vi "Initialize.vi"(7 "Serial Configuration":T1={"Baud Rate"=9600, "Parity"=0, "Data Bits"=8, "Stop Bits"=10, "Flow Control"=0} {"Flow Control" items=["None", "XON/XOFF", "RTS/CTS", "XON/XOFF & RTS/CTS", "DTR/DSR", "XON/XOFF & DTR/DSR"]; "Stop Bits" items=["1.0"=10, "1.5"=15, "2.0"=20]; "Data Bits" items=["7"=7, "8"=8]; "Parity" items=["None", "Odd", "Even", "Mark", "Space"]; "Baud Rate" items=["300"=300, "600"=600, "1200"=1200, "2400"=2400, "4800"=4800, "9600"=9600, "19200"=19200]}, 8 "error in (no error)":errorcluster, 9 "Reset (True)":bool=TRUE, 10 "ID Query (True)":bool=TRUE, 11 "VISA resource name":refnum<visa-resource-name>) -> (0 "error out":errorcluster, 3 "VISA resource name out":refnum<visa-resource-name>)   [LabVIEW 2012, in "ValveController.lvlib"]
doc: "Establishes communication with the instrument and optionally performs an instrument identification query and/or an instrument reset. It also places the instrument in a default state needed for other instrument driver operations. Therefore, call this VI before calling other instrument driver VIs for this instrument. Generally, you need to call the Initialize VI only once at the beginning of an application."
uses:
  <instrlib>/ValveController/ValveController.lvlib
panel:
  # "(c) 2007 <Enter Company Name Here>.  ALL RIGHTS RESERVED."
  # "EDIT: Change control description to remove example text for buses not supported."
  # "EDIT: Serial settings must match those on the physical instrument.  Review user's manual to determine the correct Flow Control protocol for the instrument.  \"None\" is the least robust option for this setting, and could lead to unreliable data transmission."
  # "EDIT: If your instrument does not support ID query or Reset, remove the ID Query or Reset control from the front panel and delete the case structure with the ID Query or Reset code from the block diagram."
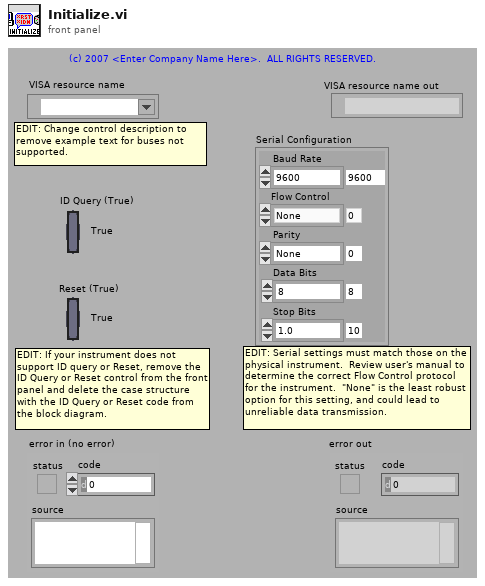
[diagram p1: front panel]
types:
  T1 = cluster{"Baud Rate":u32, "Parity":u16, "Data Bits":u16, "Stop Bits":u16, "Flow Control":u16}
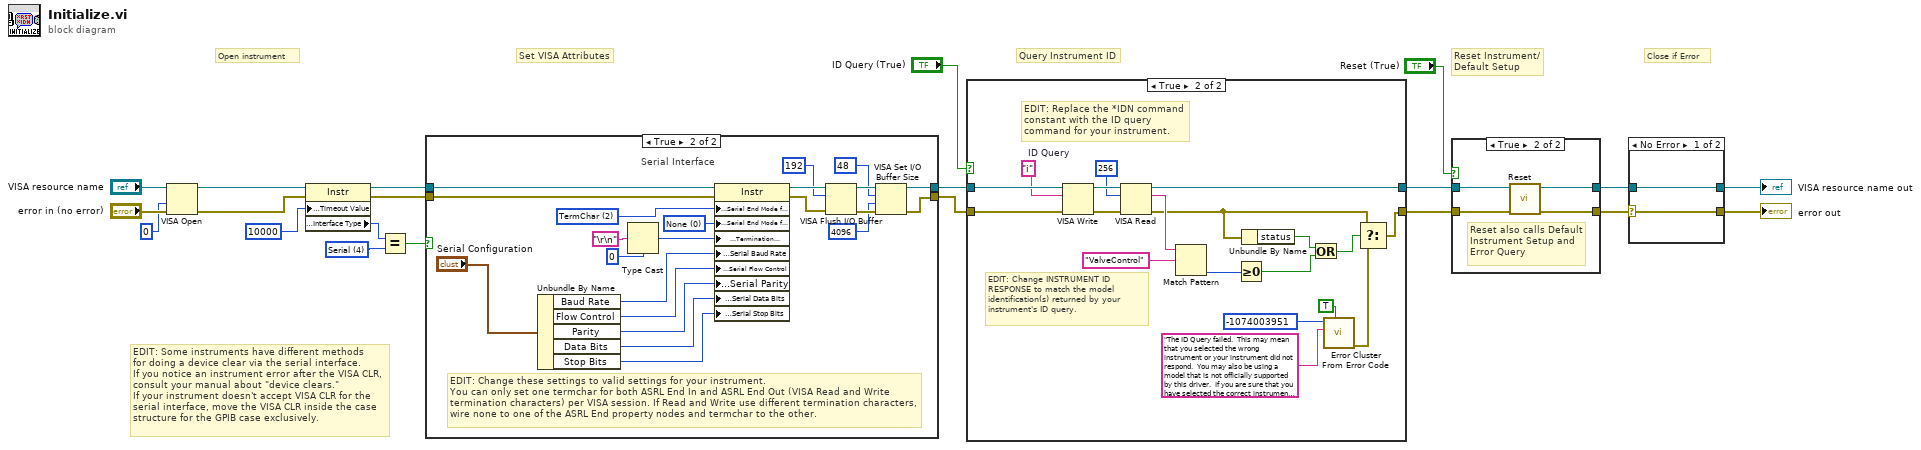
[diagram p0: block diagram]
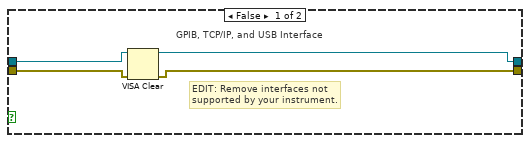
[diagram p2: hidden frame]
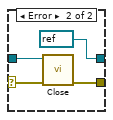
[diagram p3: hidden frame]
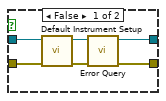
[diagram p4: hidden frame]
diagram:
  w8 = u16 4 items=["GPIB"=1, "VXI"=2, "GPIB-VXI"=3, "Serial"=4, "PXI"=5, "TCPIP"=6, "USB"=7] ("Interface Information:Interface Type")
  # "EDIT: Some instruments have different methods\nfor doing a device clear via the serial interface.  \nIf you notice an instrument error after the VISA CLR,\nconsult your manual about \"device clears.\"  \nIf your instrument doesn't accept VISA CLR for the\nserial interface, move the VISA CLR inside the case \nstructure for the GPIB case exclusively."
  # "Set VISA Attributes"
  # "Close if Error"
  # "Query Instrument ID"
  # "Reset Instrument/\nDefault Setup"
  # "Open instrument"
  n1 = VISA Open(access mode=u32 0, error in (no error)="error in (no error)", VISA resource name="VISA resource name") -> (VISA resource name=w1:refnum<visa-resource-name>, error out=w2:errorcluster)  [unwired: 2 in]
  n2 = property class="Instr"(reference=w1, error in=w2, "General Settings:Timeout Value"=u32 10000) -> (reference out=w11:refnum<visa-resource-name>, error out=w10:errorcluster, "Interface Information:Interface Type"=w15:u16)
  n3 = Equal?(x=w15, y=w8) -> (x = y?=w9:bool)
  n4 = case shown="True" w9 {
    tunnel: [w22 w44] -> w13
    tunnel: [w23 w41] -> w12
    tunnel: w11 -> [w25 w46]
    tunnel: w10 -> [w24 w47]
    frame False {
      # "EDIT: Remove interfaces not\nsupported by your instrument."
      # "GPIB, TCP/IP, and USB Interface"
      n5 = VISA Clear(VISA resource name=w25, error in (no error)=w24) -> (VISA resource name out=w22:refnum<visa-resource-name>, error out=w23:errorcluster)
    }
    frame True {
      w26 = u16 0 items=["None", "Last Bit", "TermChar", "Break"] ("Serial Settings:End Mode for Writes")
      w34 = u16 2 items=["None", "LastBit", "TermChar"] ("Serial Settings:Serial End Mode for Reads")
      # "EDIT: Change these settings to valid settings for your instrument.\nYou can only set one termchar for both ASRL End In and ASRL End Out (VISA Read and Write termination characters) per VISA session. If Read and Write use different termination characters, wire none to one of the ASRL End property nodes and termchar to the other."
      # "Serial Interface"
      n6 = Unbundle By Name("Serial Configuration") -> ("Baud Rate"=w32:u32, "Flow Control"=w28:u16, "Parity"=w30:u16, "Data Bits"=w31:u16, "Stop Bits"=w27:u16)
      n7 = Type Cast(type=u8 0, x="\r\n") -> (*(type *) &x=w33:u8)
      n8 = property class="Instr"(reference=w46, error in=w47, "Serial Settings:Serial End Mode for Reads"=w34, "Serial Settings:Serial End Mode for Writes"=w26, "Message Based Settings:Termination Character"=w33, "Serial Settings:Serial Baud Rate"=w32, "Serial Settings:Serial Flow Control"=w28, "Serial Settings:Serial Parity"=w30, "Serial Settings:Serial Data Bits"=w31, "Serial Settings:Serial Stop Bits"=w27) -> (reference out=w40:refnum<visa-resource-name>, error out=w43:errorcluster)
      n9 = VISA Flush I/O Buffer(VISA resource name=w40, mask (16)=u16 192, error in (no error)=w43) -> (VISA resource name out=w45:refnum<visa-resource-name>, error out=w42:errorcluster)
      n10 = VISA Set I/O Buffer Size(VISA resource name=w45, mask (16)=u16 48, size (4096)=u32 4096 ("size (0)"), error in (no error)=w42) -> (VISA resource name out=w44:refnum<visa-resource-name>, error out=w41:errorcluster)
    }
  }
  n11 = case shown="True" "ID Query (True)" {
    tunnel: [w48 w68] -> w20
    tunnel: [w49 w65] -> w21
    tunnel: w13 -> [w49 w66]
    tunnel: w12 -> [w48 w67]
    frame False {
    }
    frame True {
      w59 = "i"  # ID Query
      # "EDIT: Replace the *IDN command\nconstant with the ID query\ncommand for your instrument."
      # "EDIT: Change INSTRUMENT ID\nRESPONSE to match the model\nidentification(s) returned by your\ninstrument's ID query."
      n12 = VISA Write(VISA resource name=w66, write buffer=w59, error in (no error)=w67) -> (VISA resource name out=w63:refnum<visa-resource-name>, error out=w62:errorcluster)  [unwired: 1 out]
      n13 = VISA Read(VISA resource name=w63, byte count=u32 256, error in (no error)=w62) -> (VISA resource name out=w65:refnum<visa-resource-name>, read buffer=w64:string, error out=w53:errorcluster)  [unwired: 1 out]
      n14 = Match Pattern(string=w64, regular expression="ValveControl") -> (offset past match=w54:i32)  [unwired: 1 in, 3 out]
      n15 = Greater Or Equal To 0?(x=w54) -> (x >= 0?=w51:bool)
      n16 = Unbundle By Name(w53) -> ("status"=w52:bool)
      n17 = Or(x=w52, y=w51) -> (x .or. y?=w50:bool)
      n18 = call <vilib>:"Error Cluster From Error Code.vi"("show call chain? (False)"=TRUE, "error message (\"\")"="The ID Query failed.  This may mean that you selected the wrong instrument or your instrument did not respond.  You may also be using a model that is not officially supported by this driver.  If you are sure that you have selected the correct instrument and it is responding, try disabling the ID Query." ("Source (VI Name)"), "error code (0)"=-1074003951 ("Code")) -> ("error out"=w58:errorcluster)  [unwired: 6 in]
      n19 = Select(t=w53, s=w50, f=w58) -> (s? t:f=w68:errorcluster)
    }
  }
  n20 = case shown="True" "Reset (True)" {
    tunnel: w20 -> [w73 w75]
    tunnel: [w70 w78] -> w3
    tunnel: w21 -> [w74 w76]
    tunnel: [w71 w77] -> w4
    frame False {
      n21 = call <instrlib>:"Default Instrument Setup.vi"("error in (no error)"=w73, "VISA resource name"=w74) -> ("error out"=w69:errorcluster, "VISA resource name out"=w72:refnum<visa-resource-name>)  [unwired: 8 in]
      n22 = call <instrlib>:"Error Query.vi"("error in (no error)"=w69, "VISA resource name"=w72) -> ("error out"=w70:errorcluster, "VISA resource name out"=w71:refnum<visa-resource-name>)  [unwired: 8 in]
    }
    frame True {
      # "Reset also calls Default Instrument Setup and Error Query"
      n23 = call <instrlib>:"Reset.vi"("error in (no error)"=w75, "VISA resource name"=w76) -> ("error out"=w78:errorcluster, "VISA resource name out"=w77:refnum<visa-resource-name>)  [unwired: 8 in]
    }
  }
  n24 = case shown="No Error" w3 {
    selector: w3 -> [w79 w82]
    tunnel: w4 -> [w80 w83]
    tunnel: [w80 refnum<visa-resource-name> refnum ("VISA resource name out")] -> w6
    tunnel: [w79 w84] -> w5
    frame No Error {
    }
    frame Error {
      n25 = call <instrlib>:"Close.vi"("error in (no error)"=w82, "VISA resource name"=w83) -> ("error out"=w84:errorcluster)  [unwired: 9 in]
    }
  }
  "VISA resource name out" <- w6
  "error out" <- w5
